vi "PPL Builder.vi"(4 "Exclude dependent packed libraries":bool=TRUE, 6 "Version number":T1={"Major"=1, "Minor"=0, "Fix"=0, "Build"=0}, 8 "error in (no error)":errorcluster, 9 "Always Included Files":path[](array[path]), 10 "Output Directory":path, 11 "LVLIB File":path) -> (0 "error out":errorcluster, 3 "Generated Files":path[](array[path]))   [LabVIEW 2018]
uses:
  <vilib>/AppBuilder/AB_API/common/AB_API Primary Exclusions.ctl
  <vilib>/AppBuilder/AB_API/common/AB_API Version Number.ctl
panel:
  in  "Build Settings":T2={"Disconnect type definitions"=TRUE, "Remove unused polymorphic VI instances"=TRUE, "Remove unused members of project libraries"=TRUE, "Modify project library file after removing unused members"=TRUE}
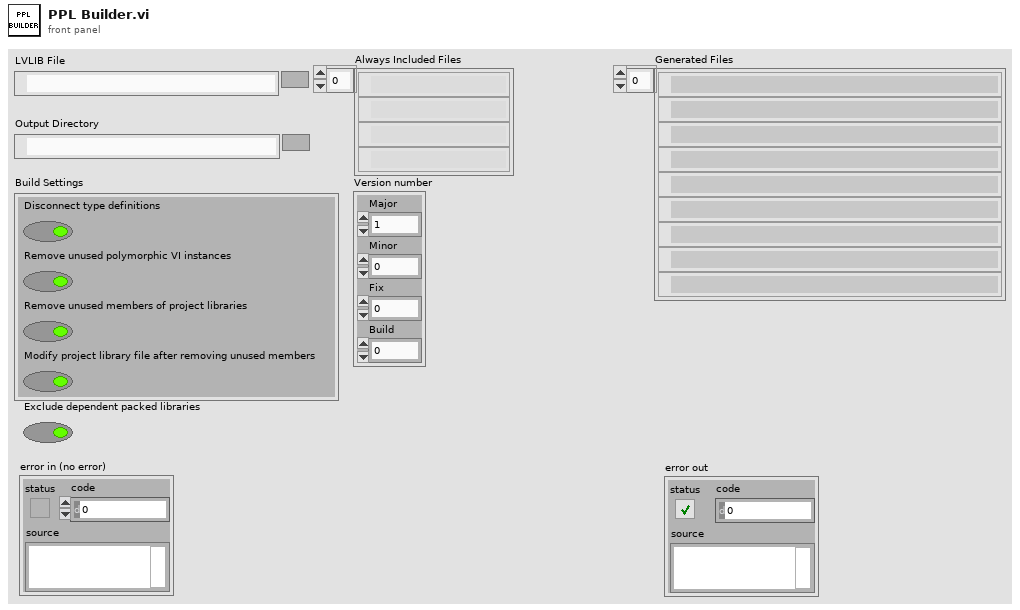
[diagram p1: front panel]
types:
  T1 = typedef "AB_API Version Number.ctl" = cluster{"Major":u16, "Minor":u16, "Fix":u16, "Build":u16}
  T2 = typedef "AB_API Primary Exclusions.ctl" = cluster{"Disconnect type definitions":bool, "Remove unused polymorphic VI instances":bool, "Remove unused members of project libraries":bool, "Modify project library file after removing unused members":bool}
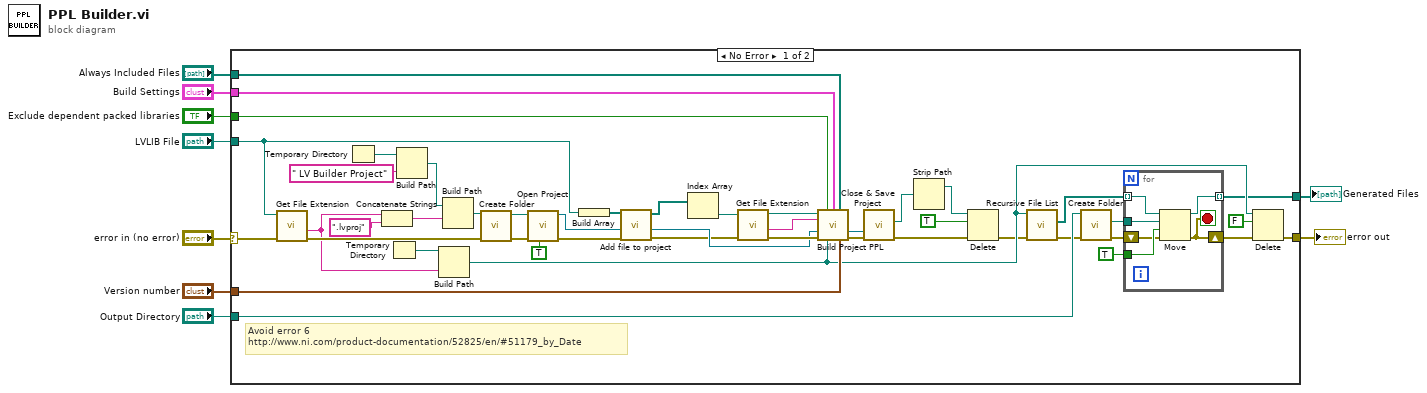
[diagram p0: block diagram]
diagram:
  n1 = case shown="No Error" "error in (no error)" {
    selector: "error in (no error)" -> [w11 w62]
    tunnel: "Build Settings" -> [w55 _]
    tunnel: "Output Directory" -> [w54 _]
    tunnel: "LVLIB File" -> [w53 _]
    tunnel: "Version number" -> [w52 _]
    tunnel: "Always Included Files" -> [w51 _]
    tunnel: "Exclude dependent packed libraries" -> [w50 _]
    tunnel: [w18 w62] -> w3
    tunnel: [w10 _] -> w1
    frame No Error {
      # "Avoid error 6\nhttp://www.ni.com/product-documentation/52825/en/#51179_by_Date"
      n2 = call <vilib>:"Get File Extension.vi"("error in (no error)"=w11, "file"=w53) -> ("error out"=w29:errorcluster, "filename without extension"=w23:string)  [unwired: 5 in, 3 out]
      n3 = Temporary Directory() -> (w12:path)
      n4 = Concatenate Strings(w23, ".lvproj" ("string")) -> (w21:string)
      n5 = Temporary Directory() -> (w20:path)
      n6 = Build Path(base path=w12, name or relative path=" LV Builder Project") -> (appended path=w25:path)
      n7 = Build Path(base path=w20, name or relative path=w23) -> (appended path=w27:path)
      n8 = Build Path(base path=w25, name or relative path=w21) -> (appended path=w24:path)
      n9 = call "Create Folder.vi"("error in (no error)"=w29, "File or Folder"=w24) -> ("error out"=w28:errorcluster, "dup File"=w13:path)  [unwired: 6 in, 2 out]
      n10 = call "Open Project.vi"("Open Window?"=TRUE, "error in (no error)"=w28, "Build Project"=w13) -> ("error out"=w49:errorcluster, "Project out"=w48:refnum<vi>)  [unwired: 7 in]
      n11 = Build Array(w53) -> (w46:path[])
      n12 = call "Add file to project.vi"("error in"=w49, "Project Ref in"=w48, "File Path"=w46) -> ("error out"=w19:errorcluster, "Project out"=w42:refnum<vi>, "Actual File Path"=w47:path[])  [unwired: 6 in]
      n13 = Index Array(array=w47) -> (element=w44:path)  [unwired: 1 in]
      n14 = call <vilib>:"Get File Extension.vi"("error in (no error)"=w19, "file"=w44) -> ("error out"=w45:errorcluster, "filename without extension"=w41:string, "dup file"=w43:path)  [unwired: 5 in, 2 out]
      n15 = call "Build Project PPL.vi"("LVLIB Path"=w43, "Exclude dependent packed libraries"=w50, "Exclusions"=w55, "Always Included Files"=w51, "Build Name"=w41, "Proj Ref"=w42, "error in (no error)"=w45, "PPL Dir"=w27, "Version number"=w52) -> ("Proj Ref Out"=w39:refnum<vi>, "error out"=w40:errorcluster)  [unwired: 3 in, 2 out]
      n16 = call "Close & Save Project.vi"("error in (no error)"=w40, "Project in"=w39) -> ("error out"=w37:errorcluster, "Path"=w16:path)  [unwired: 8 in]
      n17 = Strip Path(path=w16) -> (stripped path=w15:path)  [unwired: 1 out]
      n18 = Delete(path (use dialog)=w15, entire hierarchy (F)=TRUE, error in=w37) -> (error out=w17:errorcluster)  [unwired: 2 in, 2 out]
      n19 = call <vilib>:"Recursive File List.vi"("error in (no error)"=w17, "Folder Path"=w27) -> ("error out"=w33:errorcluster, "All Files in Dir"=w34:path[])  [unwired: 5 in, 3 out]
      n20 = call "Create Folder.vi"("error in (no error)"=w33, "File or Folder"=w54) -> ("error out"=w32:errorcluster, "Folder Path"=w31:path)  [unwired: 6 in, 2 out]
      n21 = for {
        tunnel: TRUE ("overwrite (F)") -> [w61]
        shift-right: [w57] -> w36
        shift-left: w32 -> [w60]
        tunnel: w34 -> [w59] mode=indexing
        tunnel: w31 -> [w58]
        tunnel: [w56] -> w10 mode=indexing
        stop <- w57 stop-if-true
        n22 = Move(source path=w59, error in=w60, 9:w61, 10:w58) -> (error out=w57:errorcluster, 3:w56:path)  [unwired: 1 in, 1 out]
      }
      n23 = Delete(path (use dialog)=w27, entire hierarchy (F)=FALSE ("confirm (F)"), error in=w36) -> (error out=w18:errorcluster)  [unwired: 2 in, 2 out]
    }
    frame Error {
    }
  }
  "error out" <- w3
  "Generated Files" <- w1
